vi "MCL DLL Version.vi"(8 "error in (no error)":errorcluster, 10 "revision":i16, 11 "version":i16) -> (0 "error out":errorcluster, 2 "revision out":i16, 3 "version out":i16)   [LabVIEW 2014, in "Madlib.lvlib"]
doc: "MADLIB_API void MCL_DLLVersion(short *version, short *revision);"
uses:
  <userlib>/Lambda2/lib/Madlib/Madlib.lvlib
  <userlib>/Lambda2/lib/Madlib/Madlib.dll
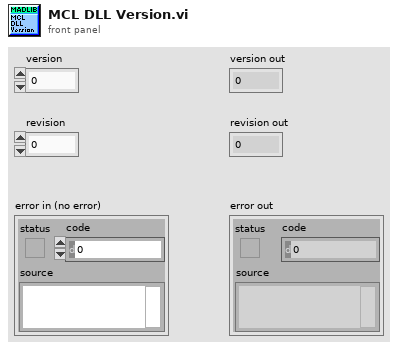
[diagram p1: front panel]
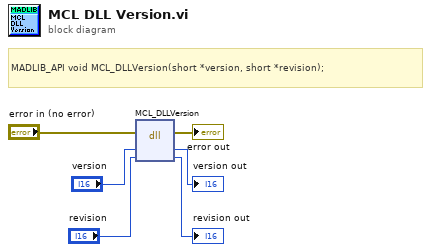
[diagram p0: block diagram]
diagram:
  # "MADLIB_API\tvoid\tMCL_DLLVersion(short *version, short *revision);"
  n1 = dll-call lib="C:/Program Files (x86)/National Instruments/LabVIEW 2014/user.lib/Lambda2/lib/Madlib/Madlib.*" fn="MCL_DLLVersion"(error in="error in (no error)", "version"="version", "revision"="revision") -> (error out=→"error out":errorcluster, "version"=→"version out":i16, "revision"=→"revision out":i16)  [unwired: 3 in, 1 out]
